vi "Parse.vi"(8 "Error In":errorcluster, 11 "object in":refnum<class "2024_18.lvclass">) -> (0 "Error Out":errorcluster, 3 "object out":refnum<class "2024_18.lvclass">)   [LabVIEW 2023, in "2024_18.lvclass"]
uses:
  2024_18.lvclass
  Common/AOC_XY(I32).ctl
  2024_18.lvclass/2024_18.ctl
  <vilib>/Utility/error.llb/Trim Whitespace One-Sided.vi
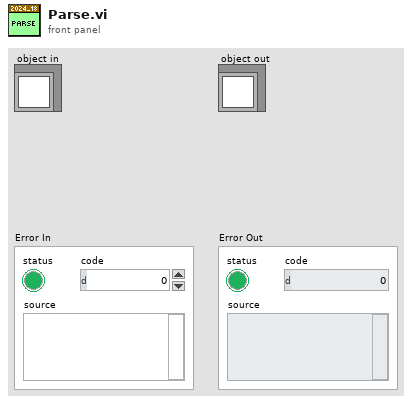
[diagram p1: front panel]
types:
  T1 = typedef "AOC_XY(I32).ctl" = cluster{"X":i32, "Y":i32}
diagram:
  (unwired) 12 ("Entries")
  (unwired) T1 {"X"=0, "Y"=0} ("XY")
  (unwired) "5,4\n4,2\n4,5\n3,0\n2,1\n6,3\n2,4\n1,5\n0,6\n3,3\n2,6\n5,1\n1,2\n5,5\n2,5\n6,5\n1,4\n0,4\n6,4\n1,1\n6,1\n1,0\n0,5\n1,6\n2,0" ("PuzzleInput")
  n1 = call <vilib>:"Trim Whitespace.vi"("string"="51,62\n23,7\n7,16\n27,12\n66,65\n51,53\n53,58\n15,21\n37,3\n20,43\n1,27\n59,40\n27,4\n25,25\n49,41\n53,46\n3,20\n56,49\n20,21\n54,37\n43,59\n61,64\n60,31\n2,1\n63,34\n31,33\n3,23\n57,54\n63,33\n59,63\n39,57\n29,9\n9,22\n59,51\n33,33\n40,51\n62,67\n51,59\n15,5\n6,3\n56,45\n16,19\n12,31\n19,2\n25,11\n23,12\n55,67\n54,43\n23,37\n41,49\n16,33\n66,43\n1,21\n22,25\n63,70\n17,26\n46,57\n56,59\n1,26\n14,29\n29,56\n10,11\n29,15\n2,17\n23,30\n13,6\n15,10\n13,12\n59,44\n15,41\n13,21\n3,17\n23,17\n17,21\n59,34\n67,59\n60,65\n15,30\n19,29\n39,63\n69,39\n19,43\n29,13\n67,51\n56,69\n63,55\n6,13\n19,3\n63,53\n59,57\n5,1\n25,32\n51,36\n44,41\n12,9\n67,68\n24,33\n55,38\n50,53\n21,11\n1,2\n35,64\n62,31\n63,61\n11,24\n47,53\n24,17\n55,55\n5,19\n65,63\n61,35\n39,68\n6,7\n64,55\n49,57\n18,23\n45,63\n32,19\n5,17\n59,64\n21,43\n46,55\n1,12\n12,15\n17,42\n68,33\n15,9\n19,30\n49,37\n29,27\n13,23\n32,31\n50,49\n64,41\n63,40\n59,61\n21,7\n25,28\n63,69\n13,35\n17,19\n27,1\n59,36\n53,64\n3,6\n30,27\n24,23\n45,60\n23,15\n69,33\n43,57\n65,31\n67,53\n46,39\n17,15\n1,13\n16,1\n55,66\n65,39\n70,35\n21,9\n41,55\n51,67\n23,28\n57,39\n57,67\n67,31\n67,60\n52,67\n19,16\n45,45\n47,66\n48,49\n59,45\n15,31\n23,23\n65,47\n9,20\n52,65\n64,59\n19,11\n66,49\n38,53\n59,49\n21,12\n49,53\n46,43\n22,1\n25,4\n62,49\n23,5\n57,41\n25,1\n19,10\n55,68\n26,61\n23,19\n21,25\n23,6\n20,25\n54,31\n27,38\n54,57\n25,26\n53,59\n2,37\n29,35\n67,35\n21,3\n27,39\n59,50\n21,29\n26,19\n25,30\n50,65\n15,22\n12,21\n63,58\n17,29\n12,1\n36,57\n6,11\n61,36\n59,53\n17,14\n55,37\n19,31\n9,17\n1,19\n33,9\n3,14\n27,22\n58,69\n17,33\n69,41\n24,35\n31,52\n51,41\n1,11\n51,65\n64,33\n53,41\n58,53\n65,62\n61,37\n24,37\n43,44\n64,61\n38,61\n1,6\n62,45\n27,27\n69,63\n35,49\n47,45\n42,55\n69,35\n50,51\n69,58\n55,65\n51,46\n15,4\n35,51\n56,35\n27,24\n45,59\n16,31\n25,10\n48,59\n23,4\n15,11\n65,43\n18,13\n17,23\n11,2\n17,5\n64,67\n13,9\n21,41\n53,49\n62,41\n25,27\n0,9\n69,69\n28,53\n63,36\n20,31\n22,7\n39,50\n51,69\n56,63\n55,35\n23,20\n19,13\n39,3\n23,42\n57,59\n59,62\n7,1\n66,47\n25,40\n54,65\n51,51\n36,53\n69,65\n52,59\n19,41\n50,61\n69,25\n7,10\n63,46\n13,1\n49,45\n12,35\n6,25\n14,9\n17,7\n23,9\n3,7\n51,56\n67,39\n49,55\n61,68\n57,42\n26,37\n1,3\n6,15\n41,46\n27,28\n21,17\n47,61\n60,33\n31,58\n43,63\n30,1\n20,35\n53,50\n13,26\n61,48\n58,49\n13,15\n15,7\n26,57\n69,31\n25,39\n0,29\n61,51\n17,22\n10,19\n21,40\n1,4\n28,7\n67,42\n13,19\n55,40\n47,44\n61,61\n59,59\n69,67\n25,23\n31,15\n30,15\n42,47\n61,66\n12,19\n17,18\n28,43\n15,27\n30,9\n3,9\n67,33\n69,45\n51,61\n22,43\n66,35\n17,12\n66,59\n69,53\n57,47\n7,23\n55,60\n63,65\n68,45\n29,32\n23,14\n67,65\n59,67\n19,24\n51,43\n19,39\n3,19\n15,13\n32,11\n34,53\n37,48\n25,8\n7,21\n29,7\n34,49\n18,5\n19,9\n64,65\n67,57\n9,23\n10,17\n47,51\n21,39\n27,33\n19,7\n14,3\n11,11\n51,55\n67,70\n9,9\n51,57\n44,65\n25,16\n19,15\n43,42\n4,5\n60,55\n12,13\n4,1\n55,70\n62,57\n11,6\n65,50\n14,23\n31,29\n41,47\n21,21\n29,3\n18,1\n25,6\n11,4\n21,27\n11,7\n60,47\n69,51\n29,10\n67,55\n37,50\n44,51\n17,17\n60,41\n19,37\n51,39\n59,39\n35,63\n52,61\n21,37\n65,69\n8,23\n8,25\n27,0\n70,55\n55,53\n67,44\n67,67\n49,61\n5,9\n7,5\n53,55\n2,13\n1,23\n69,59\n33,46\n18,33\n49,65\n21,0\n17,31\n55,69\n13,7\n61,53\n48,69\n9,1\n5,13\n8,5\n67,54\n21,30\n49,49\n14,19\n21,4\n9,15\n68,51\n15,20\n65,57\n67,52\n13,5\n0,15\n63,32\n10,25\n45,49\n3,27\n69,61\n61,49\n53,51\n41,59\n61,38\n37,7\n57,45\n21,14\n25,14\n58,43\n65,38\n14,17\n54,49\n23,25\n12,17\n55,43\n21,5\n53,47\n57,66\n27,54\n25,35\n59,31\n65,37\n20,5\n69,52\n33,3\n45,48\n11,21\n33,62\n2,19\n31,3\n6,19\n23,41\n27,41\n45,61\n26,13\n47,55\n42,59\n47,46\n1,8\n3,8\n29,29\n35,61\n65,36\n51,63\n63,49\n58,55\n69,49\n28,47\n22,15\n33,43\n56,51\n49,43\n43,51\n65,68\n29,33\n13,17\n63,51\n35,53\n1,22\n41,45\n20,3\n65,51\n5,15\n63,42\n11,13\n17,13\n58,47\n9,28\n64,51\n51,70\n23,2\n53,54\n68,67\n11,9\n14,15\n47,47\n55,63\n12,27\n43,43\n51,44\n27,8\n47,52\n17,9\n52,41\n35,59\n5,7\n2,11\n25,24\n39,53\n32,25\n3,16\n54,45\n29,30\n31,4\n56,57\n9,5\n55,51\n68,39\n13,3\n4,13\n61,43\n7,9\n37,57\n33,59\n2,25\n44,47\n57,63\n16,7\n53,45\n67,43\n49,42\n67,58\n45,53\n21,32\n23,27\n3,13\n21,18\n27,2\n55,49\n24,21\n31,31\n7,22\n15,33\n61,69\n29,1\n19,21\n14,25\n61,63\n16,11\n11,17\n3,11\n41,63\n14,35\n45,54\n1,17\n19,25\n28,35\n58,61\n48,45\n17,25\n69,64\n47,63\n50,59\n49,56\n24,41\n27,10\n70,43\n57,38\n70,69\n27,7\n24,11\n52,47\n23,39\n27,29\n1,5\n10,5\n45,47\n40,53\n65,49\n39,47\n45,57\n66,33\n19,19\n59,37\n64,45\n21,15\n10,13\n65,54\n23,38\n11,15\n55,59\n52,37\n9,31\n9,25\n61,57\n11,19\n47,57\n15,12\n50,43\n16,25\n43,41\n67,69\n67,62\n11,1\n3,1\n61,60\n41,43\n9,29\n57,32\n48,63\n19,20\n63,43\n57,61\n19,17\n63,64\n17,27\n18,17\n43,55\n66,53\n22,27\n67,56\n56,61\n52,53\n15,29\n53,65\n22,39\n32,55\n53,53\n15,17\n69,38\n48,61\n3,5\n13,25\n20,37\n4,17\n23,3\n5,11\n27,11\n57,51\n27,15\n47,41\n57,49\n17,28\n35,31\n13,39\n39,62\n69,47\n13,14\n3,43\n12,3\n33,32\n63,35\n23,13\n68,49\n58,59\n55,57\n57,56\n68,65\n50,41\n67,28\n19,35\n21,1\n29,6\n44,63\n39,56\n27,35\n21,35\n43,45\n57,69\n27,25\n59,41\n43,62\n36,63\n55,61\n6,31\n39,59\n45,55\n45,41\n15,19\n20,41\n69,55\n21,19\n15,28\n25,33\n29,51\n59,55\n19,1\n44,55\n69,34\n19,26\n61,52\n51,49\n15,6\n28,29\n49,67\n67,41\n7,8\n25,18\n48,41\n9,21\n17,11\n60,51\n15,15\n54,55\n36,3\n65,64\n13,29\n3,4\n53,61\n19,23\n7,19\n60,39\n23,26\n27,36\n44,45\n55,52\n25,9\n67,37\n39,58\n22,19\n15,3\n46,47\n21,16\n57,65\n61,59\n45,43\n8,13\n31,30\n35,3\n39,61\n40,59\n22,35\n60,43\n27,9\n15,38\n2,21\n1,9\n21,13\n41,57\n35,56\n41,53\n15,25\n23,22\n18,9\n19,27\n69,62\n35,54\n57,53\n11,5\n7,12\n37,55\n3,10\n47,59\n59,65\n11,3\n20,11\n9,16\n50,55\n45,51\n19,36\n58,65\n69,42\n9,10\n61,39\n63,39\n13,13\n54,61\n10,9\n27,3\n25,41\n13,27\n53,63\n23,29\n18,21\n39,66\n25,2\n42,41\n9,3\n65,53\n22,23\n30,5\n46,41\n21,33\n27,31\n55,48\n46,65\n19,14\n21,38\n15,23\n26,31\n17,1\n4,19\n25,29\n54,63\n4,9\n31,5\n43,39\n38,55\n69,56\n58,39\n44,57\n23,1\n68,37\n15,1\n25,15\n41,44\n29,31\n65,33\n1,7\n37,61\n5,2\n9,13\n49,47\n27,23\n65,61\n27,37\n7,20\n1,1\n47,43\n67,63\n1,15\n37,53\n5,21\n25,37\n55,54\n67,49\n65,35\n28,3\n46,63\n49,63\n49,64\n9,7\n69,57\n29,34\n25,3\n69,46\n48,53\n60,59\n13,8\n41,61\n37,63\n57,57\n3,3\n67,29\n41,62\n48,57\n17,8\n50,47\n7,17\n10,1\n53,67\n49,59\n5,5\n21,23\n61,54\n25,19\n55,39\n62,61\n52,51\n55,47\n7,6\n63,50\n38,59\n63,59\n63,63\n46,59\n41,58\n37,51\n63,52\n69,37\n5,3\n67,40\n28,59\n51,47\n36,49\n3,15\n65,59\n21,34\n16,17\n53,43\n23,11\n19,6\n25,7\n45,66\n63,37\n21,8\n65,41\n7,3\n65,48\n59,35\n17,36\n57,46\n63,47\n14,33\n9,11\n18,31\n63,41\n53,57\n59,69\n9,8\n59,47\n61,33\n45,58\n59,58\n63,57\n69,60\n47,50\n26,5\n13,31\n67,47\n62,55\n67,61\n69,48\n54,35\n46,49\n43,61\n27,26\n26,21\n22,9\n35,58\n43,60\n0,23\n8,15\n40,55\n63,38\n8,3\n29,25\n52,49\n23,35\n57,55\n19,28\n51,45\n14,1\n13,24\n69,43\n63,67\n47,65\n27,34\n55,45\n23,33\n13,11\n59,68\n65,55\n46,53\n21,31\n30,33\n8,1\n67,36\n23,31\n3,45\n4,33\n45,11\n55,26\n41,30\n35,60\n27,57\n49,26\n12,49\n38,37\n31,1\n31,62\n45,31\n0,41\n67,26\n5,31\n43,21\n43,25\n39,1\n14,65\n35,4\n1,33\n52,7\n2,43\n41,36\n52,23\n33,10\n11,44\n38,43\n63,9\n57,30\n55,17\n70,11\n19,44\n21,70\n3,52\n43,3\n47,37\n43,20\n69,9\n53,25\n3,35\n6,63\n31,25\n69,1\n44,5\n63,11\n42,15\n5,29\n11,25\n31,53\n17,58\n11,29\n45,22\n57,20\n45,27\n3,44\n17,49\n59,25\n45,14\n47,13\n33,13\n16,63\n10,41\n41,7\n29,49\n11,61\n21,57\n67,7\n61,41\n35,40\n47,6\n13,66\n55,5\n65,21\n24,45\n33,51\n63,14\n58,27\n25,60\n32,43\n29,61\n13,40\n23,54\n29,62\n24,69\n7,66\n15,36\n9,39\n53,31\n47,38\n64,3\n52,21\n1,58\n17,69\n53,13\n67,19\n36,41\n49,25\n53,7\n41,19\n4,65\n40,5\n48,21\n33,67\n59,24\n17,37\n53,30\n60,29\n11,38\n25,63\n67,11\n45,21\n61,47\n29,57\n3,24\n61,31\n42,25\n10,57\n19,66\n3,49\n51,12\n9,50\n19,61\n48,13\n39,70\n35,5\n61,65\n69,16\n35,24\n23,63\n45,5\n8,69\n24,49\n5,65\n12,55\n11,22\n47,33\n21,62\n4,41\n53,69\n22,65\n47,25\n13,69\n32,17\n30,21\n7,56\n31,35\n57,21\n31,39\n14,39\n25,57\n30,11\n51,35\n37,13\n55,23\n57,16\n57,8\n41,39\n8,29\n7,59\n19,51\n47,5\n7,39\n49,1\n51,29\n17,55\n25,53\n45,29\n51,19\n39,41\n7,67\n52,5\n10,51\n37,46\n18,45\n51,1\n13,43\n39,11\n1,55\n51,28\n39,19\n55,6\n19,52\n58,3\n56,9\n5,43\n17,38\n51,7\n31,38\n22,57\n66,5\n45,35\n3,59\n10,33\n1,47\n18,47\n19,5\n61,6\n11,52\n33,11\n66,25\n33,12\n55,15\n45,24\n13,47\n50,25\n7,49\n5,54\n37,69\n46,31\n29,5\n65,30\n10,35\n6,51\n60,1\n57,27\n39,51\n48,29\n48,15\n7,11\n53,1\n17,47\n41,66\n21,53\n25,69\n33,7\n4,29\n69,23\n31,48\n59,11\n52,33\n1,56\n64,11\n46,1\n39,7\n58,33\n43,34\n57,23\n51,33\n63,31\n43,13\n33,31\n35,19\n69,19\n49,31\n69,17\n8,51\n67,3\n53,0\n39,46\n51,2\n39,17\n31,21\n3,41\n11,69\n35,9\n37,9\n37,41\n45,3\n49,27\n14,51\n44,31\n33,53\n39,12\n39,5\n2,61\n41,64\n57,18\n42,11\n46,9\n11,67\n29,20\n3,25\n50,23\n69,4\n47,29\n15,46\n7,31\n35,69\n34,29\n24,51\n2,49\n31,47\n33,5\n40,21\n33,2\n27,58\n23,45\n9,37\n69,8\n44,69\n41,8\n33,42\n41,35\n50,7\n53,12\n35,44\n1,67\n36,37\n57,19\n33,63\n25,61\n38,31\n19,53\n63,5\n28,49\n45,6\n3,60\n5,53\n37,37\n45,20\n35,36\n33,25\n40,41\n67,14\n66,3\n27,46\n63,2\n39,39\n23,53\n63,7\n27,69\n63,29\n37,0\n23,69\n8,47\n41,65\n3,69\n38,13\n7,42\n25,59\n68,7\n34,37\n17,64\n1,65\n49,2\n1,63\n49,10\n50,33\n70,13\n17,35\n6,39\n37,33\n7,47\n57,24\n3,55\n21,59\n17,68\n51,17\n57,3\n46,11\n11,63\n49,7\n38,21\n57,31\n49,21\n63,4\n25,17\n29,60\n13,33\n59,1\n5,28\n9,30\n33,50\n41,32\n59,4\n39,16\n37,11\n13,42\n15,47\n57,29\n33,1\n11,62\n33,49\n29,26\n9,61\n5,35\n39,9\n31,13\n37,65\n43,7\n57,36\n3,57\n17,46\n22,51\n43,35\n7,37\n6,61\n36,65\n51,30\n30,37\n39,55\n45,13\n41,67\n39,37\n49,15\n19,67\n17,53\n37,39\n10,55\n4,37\n59,10\n8,33\n37,28\n19,48\n61,23\n41,23\n1,32\n9,43\n24,61\n23,46\n69,7\n62,15\n49,33\n41,2\n27,47\n47,69\n47,49\n31,16\n41,69\n15,37\n53,17\n67,15\n53,35\n25,62\n6,53\n46,27\n29,67\n68,15\n60,7\n62,17\n61,44\n49,11\n63,13\n11,41\n37,23\n27,63\n67,45\n41,13\n40,19\n3,51\n41,37\n41,34\n43,23\n55,24\n45,1\n61,12\n61,24\n39,69\n29,59\n42,29\n21,61\n23,47\n33,4\n5,36\n13,51\n36,67\n29,69\n27,56\n47,18\n31,23\n35,45\n41,3\n43,65\n7,41\n63,12\n50,37\n31,28\n54,7\n60,13\n31,65\n39,18\n51,31\n4,27\n21,55\n28,19\n5,57\n33,39\n13,63\n33,38\n61,22\n17,52\n47,39\n57,11\n57,14\n32,27\n11,28\n49,5\n36,35\n25,65\n33,29\n17,67\n19,65\n15,65\n48,3\n33,65\n51,27\n15,55\n31,67\n3,39\n53,27\n48,27\n15,45\n60,11\n57,15\n2,31\n5,27\n15,61\n37,21\n61,27\n17,51\n54,17\n67,18\n26,51\n35,15\n27,64\n57,4\n1,34\n5,48\n9,69\n1,35\n53,14\n19,50\n1,61\n27,62\n63,20\n65,44\n43,50\n21,52\n21,63\n42,69\n9,41\n35,41\n19,56\n21,48\n65,20\n13,49\n39,22\n39,32\n19,63\n52,25\n37,47\n19,69\n40,25\n51,23\n63,10\n31,41\n69,24\n31,43\n57,10\n55,1\n49,9\n37,27\n36,31\n2,41\n7,63\n3,68\n51,10\n42,35\n55,33\n11,60\n56,29\n59,21\n27,45\n64,57\n38,7\n41,31\n49,34\n8,61\n15,44\n34,13\n65,19\n43,1\n45,17\n61,67\n36,7\n35,21\n19,45\n0,49\n21,49\n27,51\n35,27\n66,9\n39,25\n63,21\n5,70\n57,35\n5,63\n61,15\n47,3\n45,15\n31,59\n43,67\n13,37\n25,49\n31,44\n19,47\n27,67\n25,45\n55,2\n51,18\n37,26\n35,39\n29,39\n39,2\n32,53\n9,54\n7,68\n28,65\n7,43\n35,23\n33,56\n49,19\n43,37\n13,46\n49,12\n7,29\n61,11\n63,19\n4,31\n21,60\n54,3\n13,44\n35,37\n69,5\n37,67\n5,52\n37,24\n43,9\n25,55\n1,37\n53,39\n9,64\n11,47\n69,22\n5,37\n34,33\n31,7\n45,25\n17,3\n22,49\n34,47\n39,13\n67,13\n21,69\n38,17\n63,3\n3,34\n23,67\n37,2\n11,59\n10,61\n25,5\n49,39\n7,46\n14,55\n67,22\n61,4\n7,57\n15,54\n29,66\n33,41\n39,14\n5,45\n35,16\n35,35\n37,35\n33,22\n35,65\n4,55\n65,15\n10,67\n62,23\n30,41\n54,19\n65,45\n13,55\n34,23\n51,3\n45,19\n37,1\n35,26\n4,25\n40,63\n41,1\n30,63\n64,21\n33,23\n13,53\n50,5\n17,45\n45,23\n23,44\n39,24\n31,9\n51,11\n62,27\n5,49\n21,67\n28,15\n27,61\n37,40\n1,60\n5,39\n37,44\n67,10\n44,33\n43,38\n49,32\n27,43\n29,12\n13,58\n53,21\n65,0\n9,33\n41,68\n31,40\n29,41\n29,47\n35,1\n29,65\n9,34\n30,19\n45,39\n32,69\n16,57\n33,55\n56,23\n29,21\n46,25\n20,57\n9,19\n40,7\n35,47\n41,40\n24,57\n46,35\n65,16\n29,58\n53,9\n67,1\n7,38\n47,67\n7,33\n6,45\n61,13\n16,41\n48,11\n62,9\n57,17\n3,37\n1,25\n65,26\n39,43\n44,1\n37,68\n59,13\n45,28\n11,33\n4,67\n38,39\n22,53\n49,69\n29,53\n17,63\n9,26\n13,61\n15,59\n63,6\n61,20\n51,13\n47,8\n5,41\n3,33\n32,21\n51,38\n35,57\n37,25\n39,45\n1,69\n12,69\n57,1\n8,43\n29,19\n7,45\n8,55\n36,13\n69,2\n21,47\n43,69\n17,43\n33,19\n4,59\n21,68\n9,55\n35,28\n33,40\n67,23\n54,15\n12,63\n38,29\n48,23\n55,25\n61,19\n17,57\n37,34\n11,37\n25,68\n5,25\n6,59\n9,59\n51,37\n25,43\n44,23\n67,21\n59,9\n13,50\n47,0\n39,35\n65,17\n67,6\n33,37\n35,7\n5,51\n17,56\n61,16\n48,67\n41,33\n28,51\n16,61\n27,40\n35,67\n3,61\n19,60\n47,21\n42,9\n33,15\n41,15\n55,29\n36,11\n68,19\n41,21\n1,46\n65,1\n41,51\n12,57\n43,27\n53,68\n3,21\n47,34\n13,68\n25,31\n65,5\n59,30\n39,23\n39,29\n5,61\n69,29\n5,68\n42,19\n13,60\n18,69\n31,11\n55,31\n39,31\n33,45\n23,65\n28,39\n55,3\n4,47\n45,36\n40,27\n57,43\n41,9\n29,23\n47,1\n26,43\n43,5\n69,13\n11,65\n35,52\n58,13\n27,53\n37,31\n42,53\n27,13\n65,13\n39,42\n29,17\n29,37\n31,8\n37,19\n15,69\n59,17\n47,19\n13,41\n43,49\n58,21\n33,47\n32,47\n53,19\n35,10\n25,70\n39,38\n49,13\n11,54\n9,53\n57,28\n38,65\n9,51\n28,23\n5,62\n5,42\n49,8\n41,11\n31,49\n33,35\n5,55\n44,27\n14,63\n7,30\n33,14\n6,33\n25,21\n56,5\n7,27\n9,36\n17,59\n27,21\n33,69\n11,23\n67,25\n33,66\n19,59\n10,69\n55,22\n11,30\n24,55\n19,57\n5,50\n61,2\n29,45\n39,15\n29,63\n23,57\n15,48\n55,18\n5,69\n31,68\n65,12\n1,51\n2,69\n3,50\n59,23\n7,55\n11,66\n23,51\n36,19\n61,1\n41,41\n16,49\n15,68\n59,19\n7,51\n31,51\n48,35\n30,55\n27,19\n1,52\n2,55\n43,14\n42,27\n27,65\n43,11\n43,30\n18,39\n61,3\n9,38\n41,16\n4,57\n43,4\n35,29\n36,15\n18,41\n30,49\n69,11\n0,39\n15,51\n11,55\n49,51\n41,5\n44,13\n56,33\n7,48\n17,34\n6,65\n37,43\n3,29\n17,41\n13,52\n69,15\n23,58\n43,31\n49,35\n15,35\n42,49\n33,27\n26,53\n69,21\n48,5\n13,45\n63,8\n39,10\n49,17\n2,29\n1,29\n51,5\n41,27\n68,11\n48,17\n21,45\n39,67\n59,27\n55,21\n51,15\n67,9\n59,15\n34,67\n26,17\n57,7\n66,19\n51,14\n3,46\n17,65\n55,19\n44,3\n3,47\n41,25\n44,37\n20,55\n14,47\n43,52\n57,25\n63,18\n5,44\n44,11\n12,37\n11,43\n9,63\n13,65\n13,67\n37,59\n49,40\n21,46\n39,48\n35,70\n31,17\n25,46\n5,59\n61,25\n55,13\n52,31\n33,17\n53,15\n38,5\n59,26\n29,11\n47,11\n59,5\n0,63\n61,55\n35,33\n15,39\n36,43\n43,29\n35,8\n57,5\n47,31\n13,59\n42,3\n1,49\n35,55\n68,31\n42,21\n7,69\n61,7\n5,67\n60,19\n65,8\n55,12\n21,65\n46,3\n7,35\n15,62\n29,16\n43,17\n53,28\n52,39\n60,15\n15,63\n21,51\n23,61\n33,61\n33,60\n52,9\n28,67\n60,27\n44,9\n59,3\n51,21\n15,66\n58,7\n17,61\n11,46\n55,27\n66,23\n39,36\n53,23\n19,54\n1,59\n59,29\n59,7\n63,27\n5,47\n26,65\n3,63\n1,39\n27,5\n43,47\n22,61\n26,49\n39,21\n50,67\n31,63\n39,65\n49,29\n23,55\n19,64\n4,23\n33,68\n47,30\n3,38\n45,18\n25,51\n20,67\n34,45\n35,18\n31,37\n39,33\n47,20\n63,26\n53,37\n11,57\n30,69\n31,14\n10,47\n45,65\n7,15\n20,63\n31,66\n32,1\n61,21\n35,6\n6,27\n34,27\n54,27\n53,33\n31,45\n14,57\n34,1\n31,19\n11,53\n35,20\n42,67\n25,67\n1,43\n35,43\n67,27\n11,45\n11,27\n56,41\n49,3\n53,4\n9,57\n45,67\n49,4\n23,59\n53,42\n3,64\n54,9\n8,63\n47,27\n23,49\n41,29\n48,37\n42,7\n65,3\n3,31\n17,39\n33,8\n33,57\n27,17\n39,49\n29,43\n3,62\n64,29\n43,53\n19,33\n53,11\n65,27\n45,9\n17,50\n35,13\n67,17\n63,1\n43,19\n11,42\n33,6\n63,25\n56,1\n61,17\n35,22\n13,57\n46,15\n40,49\n47,17\n7,7\n34,17\n9,67\n11,48\n15,49\n34,57\n9,44\n59,22\n13,32\n34,63\n68,29\n59,33\n3,67\n41,17\n35,11\n69,27\n47,23\n37,29\n31,64\n45,37\n59,18\n29,46\n35,17\n25,13\n11,31\n55,11\n62,29\n31,2\n2,35\n54,21\n65,23\n9,65\n57,13\n11,40\n9,47\n9,58\n11,49\n27,55\n33,21\n31,55\n2,65\n19,55\n65,29\n56,15\n65,28\n58,1\n64,23\n65,67\n52,1\n17,4\n61,29\n40,29\n37,45\n49,22\n57,33\n32,35\n45,7\n36,61\n67,5\n39,0\n5,23\n63,23\n50,19\n67,4\n47,15\n32,59\n15,67\n30,43\n57,9\n63,45\n63,17\n27,59\n51,9\n30,23\n61,5\n65,11\n65,7\n53,29\n54,33\n54,25\n23,64\n45,69\n39,27\n31,36\n49,23\n41,38\n31,57\n52,17\n8,39\n47,7\n37,15\n16,43\n7,13\n29,55\n47,9\n38,9\n31,24\n49,68\n27,68\n5,22\n68,1\n1,45\n70,31\n53,5\n31,61\n61,45\n7,25\n55,7\n7,65\n66,15\n50,15\n66,1\n23,21\n68,25\n41,12\n6,35\n51,20\n65,9\n6,57\n35,32\n69,3\n30,45\n57,37\n37,49\n31,69\n43,26\n24,65\n61,9\n65,65\n39,4\n19,49\n52,15\n3,65\n45,33\n23,43\n33,34\n15,53\n55,41\n9,45\n5,33\n53,3\n43,18\n9,35\n51,25\n17,54\n7,40\n9,27\n11,39\n47,35\n15,57\n65,25\n15,43\n47,24\n69,20\n23,66\n67,12\n31,27\n9,66\n37,17\n56,11\n46,69\n45,16\n19,58\n1,41\n3,53\n7,61\n25,47\n63,15\n15,60\n30,51\n27,49\n43,33\n27,42\n1,31\n17,66\n1,57\n3,40\n43,15\n1,66\n35,25\n1,53\n59,43\n7,53\n1,48\n63,24\n8,59\n42,23\n25,48\n39,34\n37,5\n11,35\n1,54\n11,51\n55,9\n40,11\n49,30\n18,61\n70,27\n9,49\n48,24\n22,16\n26,35\n22,56\n5,58\n18,7\n24,16\n17,60\n35,50\n62,39\n63,44\n25,22\n70,2\n46,24\n26,30\n0,6\n24,34\n8,32\n40,12\n62,12\n40,33\n10,65\n26,41\n18,55\n50,22\n42,2\n32,9\n30,61\n14,2\n9,56\n15,18\n58,35\n36,20\n70,48\n36,18\n28,8\n64,63\n26,15\n70,36\n21,50\n22,2\n64,15\n63,56\n34,24\n16,42\n48,26\n61,62\n50,16\n51,42\n38,18\n54,56\n7,60\n68,38\n57,26\n31,26\n2,58\n24,68\n69,18\n50,17\n13,0\n10,18\n53,22\n68,2\n28,2\n26,39\n28,34\n46,17\n42,32\n34,39\n32,44\n60,25\n33,16\n24,31\n4,24\n38,11\n42,17\n14,58\n54,1\n43,2\n42,6\n20,64\n44,61\n20,48\n20,51\n28,31\n67,32\n4,28\n40,9\n66,57\n24,3\n53,18\n46,2\n2,20\n23,70\n26,9\n58,34\n59,20\n42,5\n8,64\n58,36\n0,1\n40,34\n60,17\n30,4\n62,44\n40,22\n60,20\n65,34\n44,2\n48,51\n22,62\n48,4\n38,26\n32,49\n69,40\n31,18\n66,42\n32,50\n41,20\n31,0\n56,8\n60,26\n46,16\n57,12\n53,44\n0,70\n38,28\n22,29\n40,24\n24,8\n37,12\n44,29\n44,34\n66,27\n28,52\n24,39\n28,27\n8,53\n36,39\n64,24\n30,38\n56,16\n33,28\n32,51\n26,10\n14,46\n4,7\n30,47\n64,37\n60,36\n31,42\n44,0\n46,54\n32,14\n36,8\n32,40\n20,1\n37,64\n63,0\n34,16\n21,42\n46,21\n56,2\n69,32\n62,19\n29,18\n49,6\n62,1\n40,23\n70,10\n46,18\n42,34\n50,38\n24,42\n70,58\n66,11\n45,4\n22,64\n36,64\n20,46\n68,32\n53,34\n69,28\n36,36\n2,59\n70,44\n65,40\n24,19\n11,0\n14,69\n34,19\n19,8\n66,44\n45,32\n22,42\n24,36\n0,37\n38,15\n4,70\n3,70\n44,10\n0,48\n24,25\n56,21\n68,8\n58,31\n21,2\n48,68\n41,4\n21,26\n56,18\n18,22\n10,64\n62,43\n55,32\n66,0\n40,3\n70,46\n23,24\n62,13\n20,29\n48,6\n47,32\n48,0\n64,28\n34,15\n50,42\n60,42\n22,32\n69,36\n60,14\n20,7\n17,44\n70,28\n18,2\n44,40\n60,3\n16,59\n8,20\n50,18\n8,57\n66,34\n20,36\n20,54\n21,64\n65,2\n0,46\n64,20\n12,58\n18,0\n38,30\n36,16\n70,8\n6,32\n64,17\n30,6\n62,2\n36,40\n68,17\n44,14\n45,8\n6,64\n20,65\n43,36\n57,2\n54,30\n40,35\n66,16\n70,26\n44,16\n39,26\n4,32\n42,0\n59,38\n42,26\n44,58\n64,49\n60,4\n29,44\n50,26\n43,28\n18,59\n48,10\n24,52\n42,66\n26,26\n68,6\n66,32\n27,16\n10,68\n52,38\n50,31\n59,8\n26,70\n8,19\n48,55\n28,18\n54,24\n65,46\n70,1\n2,32\n51,52\n55,50\n13,64\n62,33\n60,5\n64,48\n22,28\n2,57\n12,60\n58,6\n34,43\n24,56\n14,66\n34,18\n56,54\n61,42\n56,52\n41,52\n32,18\n38,41\n3,56\n28,36\n47,16\n36,10\n37,32\n45,30\n66,30\n29,48\n11,64\n60,61\n64,43\n16,64\n40,32\n70,61\n2,12\n30,36\n66,31\n29,38\n24,2\n25,12\n58,12\n6,9\n42,56\n0,5\n14,68\n24,24\n61,28\n48,38\n70,15\n60,34\n52,56\n66,46\n58,52\n23,48\n32,26\n16,62\n34,10\n45,38\n60,0\n66,24\n21,66\n20,45\n9,62\n22,52\n38,6\n26,33\n20,66\n39,52\n8,38\n34,44\n6,56\n66,6\n70,14\n66,56\n46,68\n70,16\n68,48\n67,34\n62,4\n34,30\n18,56\n32,42\n16,5\n64,12\n43,58\n42,1\n50,36\n62,22\n54,32\n26,4\n40,40\n39,44\n12,65\n29,28\n32,15\n9,0\n24,30\n42,68\n30,14\n10,60\n56,36\n47,4\n66,40\n70,24\n30,40\n56,25\n36,34\n23,18\n0,19\n50,3\n12,14\n70,47\n22,40\n14,40\n56,34\n61,10\n52,45\n46,29\n42,12\n47,2\n56,28\n42,33\n59,46\n7,64\n62,30\n48,36\n43,12\n23,0\n56,39\n24,48\n61,14\n56,27\n8,21\n24,29\n36,32\n13,56\n45,56\n42,37\n56,22\n2,70\n67,16\n56,37\n46,14\n26,69\n28,32\n25,52\n23,32\n54,36\n37,8\n22,70\n32,36\n50,6\n44,68\n47,56\n24,67\n22,69\n38,22\n2,38\n18,48\n48,16\n54,2\n46,26\n56,60\n50,39\n50,50\n16,6\n36,12\n35,42\n35,48\n66,14\n28,41\n46,7\n49,54\n22,22\n38,2\n29,40\n70,65\n66,58\n40,8\n66,55\n30,52\n38,3\n6,36\n46,45\n40,64\n2,4\n0,13\n20,60\n26,52\n48,1\n54,47\n49,70\n70,40\n54,26\n70,6\n18,4\n28,58\n10,8\n26,62\n10,38\n6,44\n4,10\n26,42\n51,68\n5,20\n70,0\n32,61\n11,18\n58,44\n36,68\n58,60\n47,22\n16,67\n30,60\n22,44\n70,32\n8,12\n46,6\n66,61\n67,24\n56,62\n20,20\n18,46\n28,1\n59,32\n24,43\n2,16\n12,16\n29,22\n18,52\n18,35\n57,58\n4,60\n64,7\n31,10\n20,68\n51,24\n64,10\n20,61\n68,22\n12,44\n20,58\n8,24\n14,36\n30,20\n41,48\n38,70\n20,13\n27,6\n9,14\n12,30\n22,20\n24,20\n62,10\n68,56\n70,4\n35,68\n26,67\n20,50\n40,15\n26,24\n40,67\n19,34\n4,64\n63,16\n61,30\n60,37\n34,35\n36,23\n41,60\n60,62\n0,53\n8,40\n10,15\n59,42\n50,63\n46,19\n60,22\n0,7\n2,39\n52,63\n22,63\n21,54\n4,4\n2,8\n20,8\n8,27\n62,69\n2,53\n6,18\n65,10\n45,0\n27,30\n45,50\n6,5\n4,3\n30,30\n61,18\n64,69\n8,60\n11,36\n66,62\n8,31\n64,68\n33,52\n54,41\n29,42\n16,44\n36,17\n34,66\n50,57\n32,48\n4,63\n54,53\n19,32\n3,18\n49,44\n4,35\n20,59\n68,26\n62,62\n46,23\n52,14\n45,2\n69,30\n67,48\n62,18\n43,46\n4,18\n12,24\n53,60\n28,25\n38,4\n50,30\n62,52\n18,24\n16,30\n66,64\n60,16\n14,0\n39,20\n59,54\n34,20\n43,64\n26,20\n33,44\n6,41\n57,64\n0,51\n48,8\n58,8\n54,52\n30,26\n56,26\n44,19\n16,8\n70,66\n58,68\n46,12\n52,32\n68,57\n48,20\n46,52\n66,39\n8,9\n33,0\n18,63\n52,60\n52,35\n68,47\n31,12\n38,14\n34,34\n18,18\n40,6\n56,0\n34,21\n35,62\n63,28\n42,28\n30,62\n5,30\n28,57\n58,18\n39,30\n1,16\n58,0\n25,34\n19,0\n34,56\n18,62\n14,21\n6,29\n49,0\n64,5\n70,30\n0,47\n60,40\n39,60\n55,62\n2,14\n50,9\n30,42\n44,21\n52,29\n23,68\n48,2\n27,50\n28,42\n4,22\n40,57\n17,6\n0,55\n54,13\n68,23\n50,48\n38,47\n56,13\n9,12\n57,34\n8,70\n4,48\n4,15\n64,54\n68,68\n58,26\n20,26\n55,42\n22,12\n41,18\n68,12\n56,3\n60,69\n52,12\n24,6\n24,53\n16,40\n20,24\n2,52\n10,59\n37,56\n4,0\n24,32\n39,28\n42,58\n51,4\n28,16\n68,59\n68,35\n24,28\n52,68\n40,20\n11,8\n7,18\n62,0\n64,1\n21,58\n38,50\n24,50\n43,22\n26,45\n54,11\n26,23\n16,18\n32,68\n42,22\n55,58\n0,14\n50,66\n5,38\n44,7\n21,44\n50,62\n2,68\n29,50\n54,12\n30,2\n56,48\n46,70\n8,34\n70,7\n56,53\n46,64\n40,0\n28,61\n14,50\n22,67\n4,8\n6,50\n32,13\n60,12\n41,26\n58,23\n31,20\n60,24\n15,58\n69,10\n20,12\n70,52\n62,32\n40,1\n39,64\n40,58\n66,29\n29,68\n18,12\n6,30\n64,50\n70,25\n6,58\n52,54\n58,37\n48,19\n4,6\n12,46\n22,30\n8,10\n26,28\n58,51\n12,11\n36,2\n32,56\n70,34\n30,7\n1,28\n30,17\n18,34\n34,42\n22,4\n18,10\n49,48\n46,34\n8,18\n56,67\n32,58\n34,11\n16,45\n20,40\n7,2\n54,20\n42,57\n37,52\n1,44\n17,48\n11,68\n9,32\n64,64\n12,45\n56,66\n58,46\n15,8\n2,34\n34,46\n18,19\n28,24\n70,51\n22,50\n26,56\n56,19\n5,34\n64,16\n11,26\n24,64\n52,8\n58,2\n20,10\n53,40\n40,43\n15,32\n29,64\n68,69\n50,44\n56,43\n5,32\n52,36\n22,47\n42,36\n16,20\n51,26\n0,65\n64,58\n8,62\n48,65\n58,17\n26,36\n18,40\n8,58\n64,38\n12,10\n51,34\n16,2\n68,3\n52,34\n0,40\n42,18\n34,54\n59,12\n2,9\n10,24\n40,13\n26,32\n38,49\n0,26\n68,42\n62,63\n54,34\n66,38\n43,68\n38,57\n52,43\n2,28\n40,30\n36,26\n11,70\n52,4\n44,62\n14,53\n4,66\n44,44\n21,6\n50,68\n26,29\n34,58\n9,42\n10,46\n46,0\n22,38\n16,46\n6,2\n43,48\n49,60\n0,25\n14,27\n56,30\n30,29\n63,30\n32,10\n30,8\n40,36\n58,24\n51,64\n62,8\n18,42\n64,47\n0,18\n70,17\n23,16\n42,62\n6,42\n14,62\n44,12\n12,8\n32,45\n12,41\n14,54\n29,54\n0,61\n27,60\n6,28\n66,8\n57,70\n28,66\n4,34\n50,20\n14,5\n52,57\n17,10\n54,8\n52,40\n8,11\n18,26\n10,10\n42,10\n16,47\n57,44\n27,18\n25,38\n66,70\n10,34\n24,15\n64,56\n36,9\n68,58\n2,50\n2,10\n65,52\n38,66\n31,46\n48,47\n44,43\n38,69\n11,50\n4,68\n42,14\n49,50\n16,68\n32,32\n25,58\n50,11" ("PuzzleInput")) -> ("trimmed string"=w13:string)  [unwired: 1 in]
  n2 = Spreadsheet String To Array(delimiter (Tab)=",", format string="%d", spreadsheet string=w13, array type (2D Dbl)=i32[][] []) -> (array=w9:i32[][])
  n3 = for {
    tunnel: [w21] -> w7 mode=indexing
    tunnel: w9 -> [w19] mode=indexing
    n4 = Index Array(array=w19) -> (element #1=w18:i32, element #2=w17:i32)  [unwired: 2 in]
    n5 = Bundle(cluster=T1 {"X"=0, "Y"=0} ("XY"), "X"=w18, "Y"=w17) -> (w21:T1)
  }
  n6 = Array Max & Min(array=w9) -> (max value=w4:i32)  [unwired: 3 out]
  n7 = Bundle(cluster=T1 {"X"=0, "Y"=0} ("XY"), "X"=w4, "Y"=w4) -> (w3:T1)
  n8 = Increment(x=w4) -> (x+1=w8:i32)
  n9 = Bundle By Name(cluster="object in", "Items"=w7, "Start"=T1 {"X"=0, "Y"=0}, "End"=w3, "Width"=w8, "Height"=w8, "Entries"=1024) -> (→"object out":refnum<class "2024_18.lvclass">)
  "Error Out" <- "Error In"
